vi "date check.vi"(8 "error in (no error)":errorcluster, 9 "month3":u16, 10 "month2":u16, 11 "month1":u16) -> (0 "error out":errorcluster)   [LabVIEW 2015, in "SCANalone4x64.lvlib"]
doc: "__declspec(dllimport) void __stdcall date_check(unsigned short month1, unsigned short month2, unsigned short month3);"
uses:
  <userlib>/SCANalone4x64/SCANalone4x64.lvlib
  <userlib>/SCANalone4x64/SCANalone4x64.dll
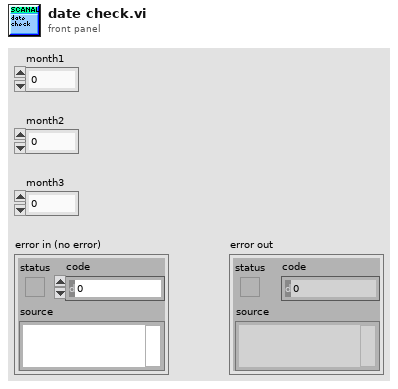
[diagram p1: front panel]
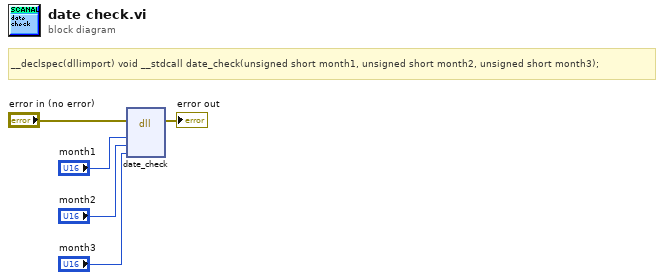
[diagram p0: block diagram]
diagram:
  # "__declspec(dllimport) void __stdcall date_check(unsigned short month1, unsigned short month2, unsigned short month3);"
  n1 = dll-call lib="C:/Program Files/National Instruments/LabVIEW 2015/user.lib/SCANalone4x64/SCANalone4x64.*" fn="date_check"(error in="error in (no error)", "month1"="month1", "month2"="month2", "month3"="month3") -> (error out=→"error out":errorcluster)  [unwired: 6 in, 1 out]
